vi "disableSCurve.vi"(0 "ACESDEController in":refnum<class "ACESDEController.lvclass">, 2 "axis (nc - for use only with multi-axis applications)":T1, 5 "error in (no error)":errorcluster) -> (14 "ACESDEController out":refnum<class "ACESDEController.lvclass">, 17 "success?":bool, 18 "response":string, 19 "error out":errorcluster)   [LabVIEW 2013, in "classes.lvlib" / "ACESDEController.lvclass"]
uses:
  ACESDEController.lvclass
  common/controls/axis.ctl
  Controller/_Controller.lvclass
  libraries/common.lvlib
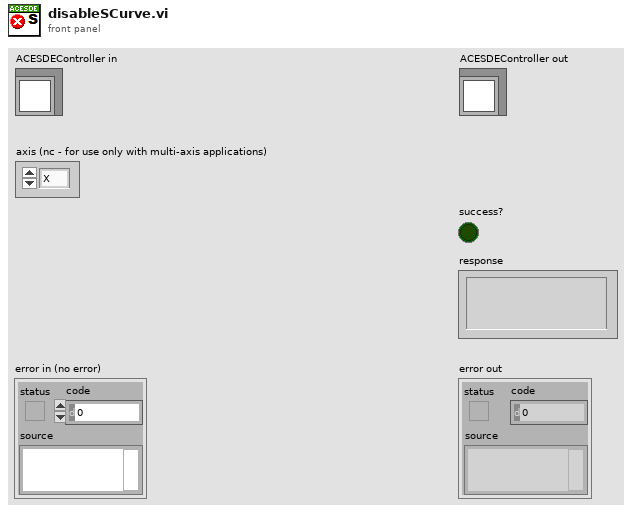
[diagram p1: front panel]
types:
  T1 = typedef "common.lvlib/axis.ctl" = enum16{"X", "Y", "Z", "U"}
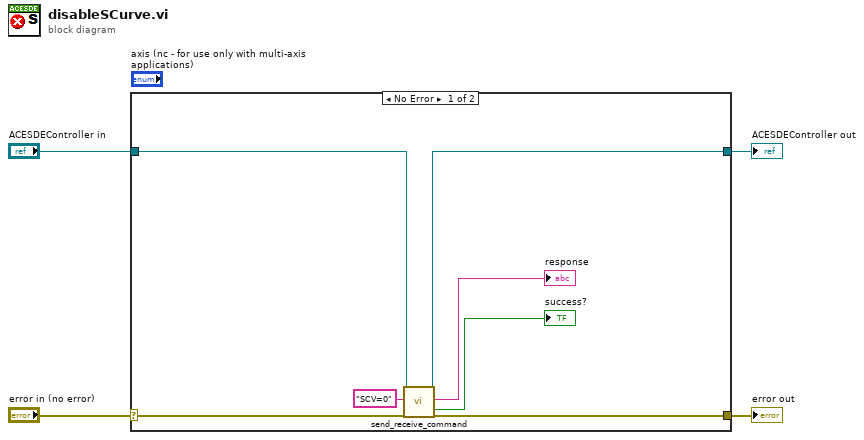
[diagram p0: block diagram]
diagram:
  n1 = case shown="No Error" "error in (no error)" {
    selector: "error in (no error)" -> [w8 w13]
    tunnel: [w7 w13] -> w3
    tunnel: [w5 w12] -> w1
    tunnel: "ACESDEController in" -> [w6 w12]
    frame No Error {
      n2 = call "send_receive_command.vi"("reference (in)"=w6, "ASCII Command (in)"="SCV=0", "error in (no error)"=w8) -> ("reference (out)"=w5:refnum<class "ACESDEController.lvclass">, "response (out)"=→"response":string, "success?"=→"success?":bool, "error out"=w7:errorcluster)  [unwired: 12 in, 1 out]
    }
    frame Error {
    }
  }
  "error out" <- w3
  "ACESDEController out" <- w1
